vi "AmplitudeArray.vi"(4 "NLEIS Run Mode":bool caption="Test        Sweep", 5 "Test Amplitude (mA)":dbl, 6 "Amplitude\nArray Source":bool, 7 "Manual Amplitudes":dbl[](array[numeric]), 8 "# Amplitudes (Manual)":i32, 9 "Smallest Amplitude (mA)":dbl=1.0 format="%#.6f", 10 "Largest Amplitude (mA)":dbl=1.0 format="%#.5f", 11 "# Amplitudes (Auto)":i32=20) -> (2 "Amplitudes (A)":dbl[](array[numeric]), 3 "# Amplitudes":i32)   [LabVIEW 2018]
panel:
  # "Input"
  # "Output"
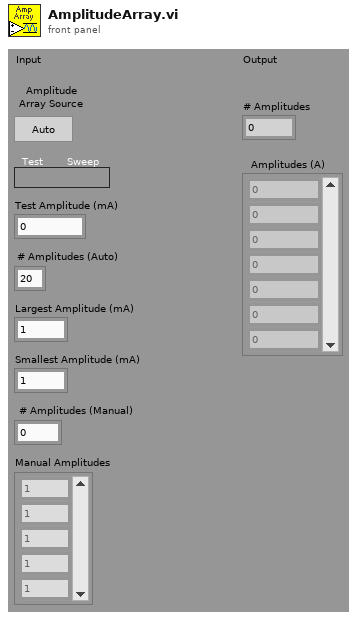
[diagram p1: front panel]
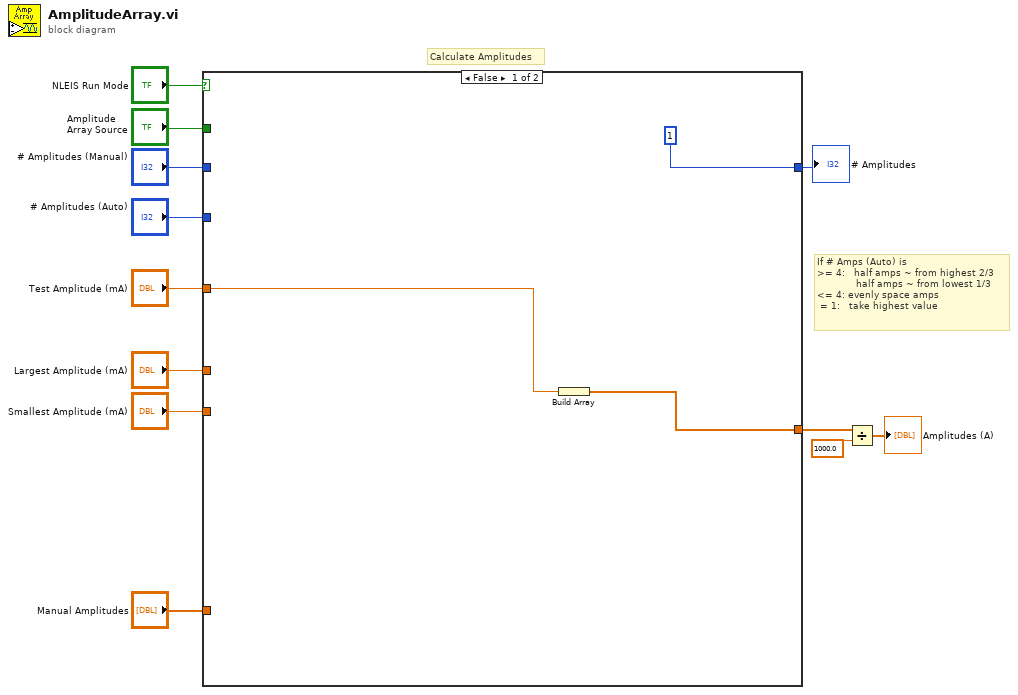
[diagram p0: block diagram]
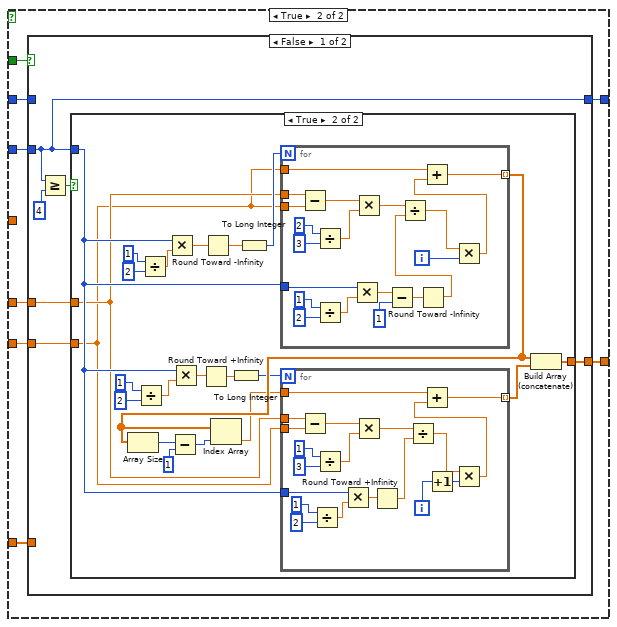
[diagram p2: hidden frame]
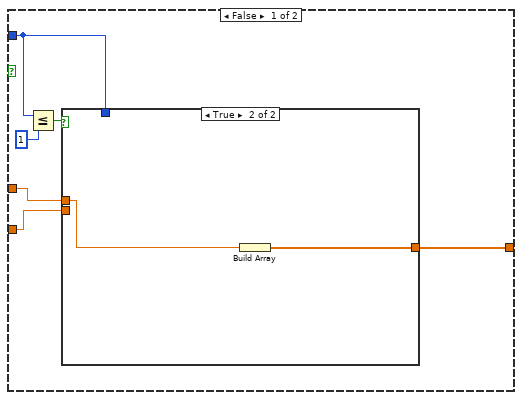
[diagram p3: hidden frame]
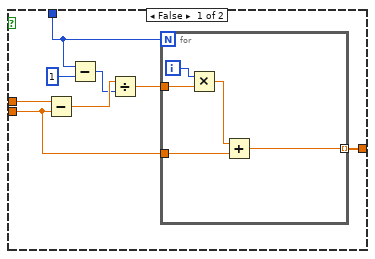
[diagram p4: hidden frame]
diagram:
  # "If # Amps (Auto) is\n>= 4:   half amps ~ from highest 2/3\n             half amps ~ from lowest 1/3\n<= 4: evenly space amps\n = 1:   take highest value"
  # "Calculate Amplitudes"
  n1 = case shown="False" "NLEIS Run Mode" {
    tunnel: [w14 w23] -> w2
    tunnel: [1 w22] -> w11
    tunnel: "Amplitude\nArray Source" -> [_ w21]
    tunnel: "# Amplitudes (Auto)" -> [_ w20]
    tunnel: "# Amplitudes (Manual)" -> [_ w19]
    tunnel: "Test Amplitude (mA)" -> [w13 _]
    tunnel: "Manual Amplitudes" -> [_ w18]
    tunnel: "Largest Amplitude (mA)" -> [_ w17]
    tunnel: "Smallest Amplitude (mA)" -> [_ w16]
    frame False {
      n2 = Build Array(w13) -> (w14:dbl[])
    }
    frame True {
      n3 = case shown="False" w21 {
        tunnel: [w29 w112] -> w23
        tunnel: [w25 w113] -> w22
        tunnel: w20 -> [w25 _]
        tunnel: w19 -> [_ w113]
        tunnel: w18 -> [_ w112]
        tunnel: w17 -> [w28 _]
        tunnel: w16 -> [w27 _]
        frame False {
          n4 = Greater Or Equal?(x=w25, y=4) -> (x >= y?=w26:bool)
          n5 = case shown="True" w26 {
            tunnel: [w33 w72] -> w29
            tunnel: w25 -> [w31 w53]
            tunnel: w28 -> [w35 w52]
            tunnel: w27 -> [w34 w51]
            frame False {
              n6 = Less Or Equal?(x=w31, y=1) -> (x <= y?=w30:bool)
              n7 = case shown="True" w30 {
                tunnel: w35 -> [w43 w50]
                tunnel: w34 -> [w41 _]
                tunnel: [w39 w49] -> w33
                tunnel: w31 -> [w37 _]
                frame False {
                  n8 = Subtract(x=w43, y=w41) -> (x-y=w42:dbl)
                  n9 = Subtract(x=w37, y=1) -> (x-y=w36:i32)
                  n10 = Divide(x=w42, y=w36) -> (x/y=w40:dbl)
                  n11 = for {
                    N: w37 -> [_]
                    tunnel: w41 -> [w48]
                    tunnel: w40 -> [w47]
                    tunnel: [w44] -> w39 mode=indexing
                    i -> [w46]
                    n12 = Multiply(x=w46, y=w47) -> (x*y=w45:dbl)
                    n13 = Add(x=w45, y=w48) -> (x+y=w44:dbl)
                  }
                }
                frame True {
                  n14 = Build Array(w50) -> (w49:dbl[])
                }
              }
            }
            frame True {
              n15 = Divide(x=1, y=2) -> (x/y=w66:dbl)
              n16 = Divide(x=1, y=2) -> (x/y=w69:dbl)
              n17 = Multiply(x=w53, y=w69) -> (x*y=w55:dbl)
              n18 = Multiply(x=w53, y=w66) -> (x*y=w61:dbl)
              n19 = Round Toward +Infinity(x=w61) -> (ceil(x): smallest int >= x=w62:dbl)
              n20 = Round Toward -Infinity(1:w55) -> (0:w64:dbl)
              n21 = To Long Integer(number=w62) -> (32bit integer=w60:i32)
              n22 = To Long Integer(number=w64) -> (32bit integer=w63:i32)
              n23 = for {
                N: w63 -> [_]
                tunnel: w53 -> [w94]
                tunnel: [w100] -> w65 mode=indexing
                tunnel: w52 -> [w99]
                tunnel: w51 -> [w98]
                tunnel: w51 -> [w97]
                i -> [w102]
                n24 = Subtract(x=w99, y=w98) -> (x-y=w110:dbl)
                n25 = Divide(x=2, y=3) -> (x/y=w109:dbl)
                n26 = Divide(x=1, y=2) -> (x/y=w105:dbl)
                n27 = Multiply(x=w94, y=w105) -> (x*y=w96:dbl)
                n28 = Multiply(x=w110, y=w109) -> (x*y=w104:dbl)
                n29 = Subtract(x=w96, y=1) -> (x-y=w93:dbl)
                n30 = Round Toward -Infinity(1:w93) -> (0:w92:dbl)
                n31 = Divide(x=w104, y=w92) -> (x/y=w103:dbl)
                n32 = Multiply(x=w103, y=w102) -> (x*y=w101:dbl)
                n33 = Add(x=w97, y=w101) -> (x+y=w100:dbl)
              }
              n34 = Array Size(array=w65) -> (size(s)=w57:i32)
              n35 = Subtract(x=w57, y=1) -> (x-y=w58:i32)
              n36 = Index Array(array=w65, index=w58) -> (element=w59:dbl)
              n37 = for {
                N: w60 -> [_]
                tunnel: [w85] -> w54 mode=indexing
                tunnel: w52 -> [w84]
                tunnel: w51 -> [w83]
                tunnel: w59 -> [w82]
                tunnel: w53 -> [w75]
                i -> [w74]
                n38 = Subtract(x=w84, y=w83) -> (x-y=w90:dbl)
                n39 = Divide(x=1, y=2) -> (x/y=w78:dbl)
                n40 = Divide(x=1, y=3) -> (x/y=w89:dbl)
                n41 = Multiply(x=w75, y=w78) -> (x*y=w77:dbl)
                n42 = Multiply(x=w90, y=w89) -> (x*y=w88:dbl)
                n43 = Round Toward +Infinity(x=w77) -> (ceil(x): smallest int >= x=w76:dbl)
                n44 = Divide(x=w88, y=w76) -> (x/y=w87:dbl)
                n45 = Increment(x=w74) -> (x+1=w73:i32)
                n46 = Multiply(x=w87, y=w73) -> (x*y=w86:dbl)
                n47 = Add(x=w82, y=w86) -> (x+y=w85:dbl)
              }
              n48 = Build Array (concatenate)(w65, w54) -> (w72:dbl[])
            }
          }
        }
        frame True {
        }
      }
    }
  }
  "# Amplitudes" <- w11
  n49 = Divide(x=w2, y=1000.0) -> (x/y=→"Amplitudes (A)":dbl[])
